vi "Prettify Class Name.vi"(9 "Class":refnum<class>) -> (1 "Pretty Class Name":string)   [LabVIEW 2020, in "IDatabase.lvlib"]
uses:
  IDatabase/IDatabase.lvlib
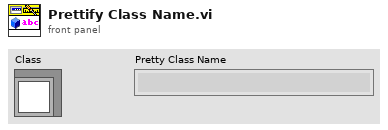
[diagram p1: front panel]
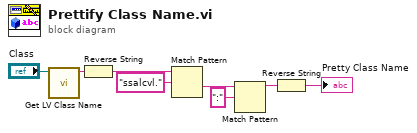
[diagram p0: block diagram]
diagram:
  n1 = call <vilib>:"Get LV Class Name.vi"("object"="Class") -> ("class name"=w8:string)  [unwired: 9 in, 1 out]
  n2 = Reverse String(1:w8) -> (0:w7:string)
  n3 = Match Pattern(string=w7, regular expression="ssalcvl.") -> (after substring=w5:string)  [unwired: 1 in, 3 out]
  n4 = Match Pattern(string=w5, regular expression=":") -> (before substring=w3:string)  [unwired: 1 in, 3 out]
  n5 = Reverse String(1:w3) -> (0:→"Pretty Class Name":string)
